vi "Unflatten Odometry Data.vi"(10 "Odometry Data":dbl[](array[numeric])) -> (1 "Heading":dbl, 2 "(X,Y) Position":dbl[](array[numeric]))   [LabVIEW 2017]
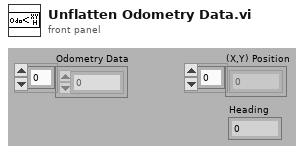
[diagram p1: front panel]
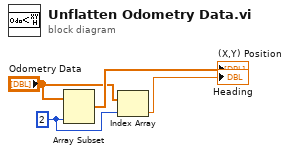
[diagram p0: block diagram]
diagram:
  w2 = 2 ("length")
  n1 = Array Subset(array="Odometry Data", length=w2) -> (→"(X,Y) Position":dbl[])  [unwired: 1 in]
  n2 = Index Array(array="Odometry Data", index=w2) -> (element=→"Heading":dbl)
